vi "Interfaz.vi"() -> ()   [LabVIEW 2023]
uses:
  <vilib>/Instr/_visa.llb/VISA Configure Serial Port (Instr).vi
panel:
  out "Real Altitude":T1(graph)
  out "Y":dbl(knob) scale=-180.0..180.0
  out "Gyro z":T1(graph)
  out "Gyro y":T1(graph)
  out "Gyro x":T1(graph)
  out "X":dbl(knob) scale=-180.0..180.0
  out "Thermometer":dbl(slide) scale=0.0..60.0
  out "salida de x":dbl[](array[numeric])
  out "Input":string
  in  "Select a file":path
  out "Barometer":T1(graph)
  out "Altitude":T1(graph)
  out "Accelerometer Z":cluster{i32[], dbl[]}(graph)
  out "Accelerometer Y":cluster{i32[], dbl[]}(graph)
  out "#Satellites":dbl
  out "Longitude":dbl
  out "Latitude":dbl
  out "Temperature":T1(graph)
  out "Accelerometer X":cluster{i32[], "output array":dbl[]}(graph)
  in  "stop":bool
  in  "Select a communication port":refnum<visa-resource-name>
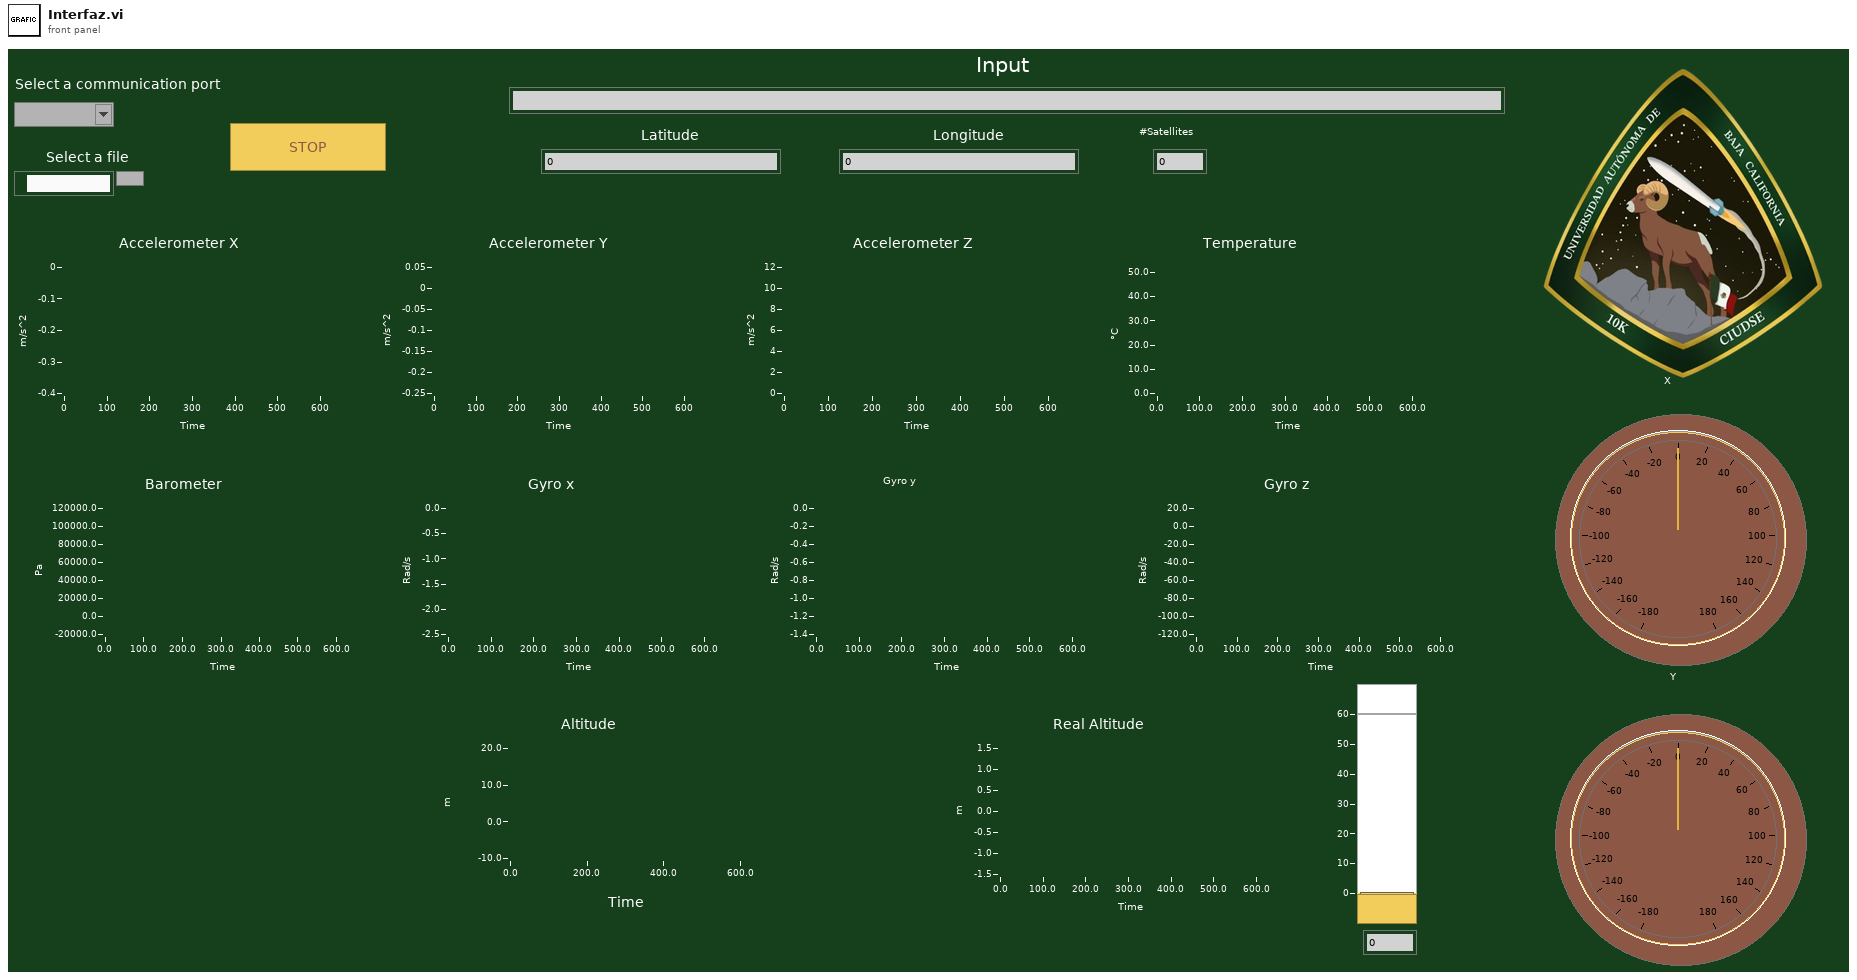
[diagram p1: front panel]
types:
  T1 = cluster{"output array":dbl[], "output array":dbl[]}
  T2 = enum16{"open", "replace", "create", "open or create", "replace or create", "replace or create with confirmation"}
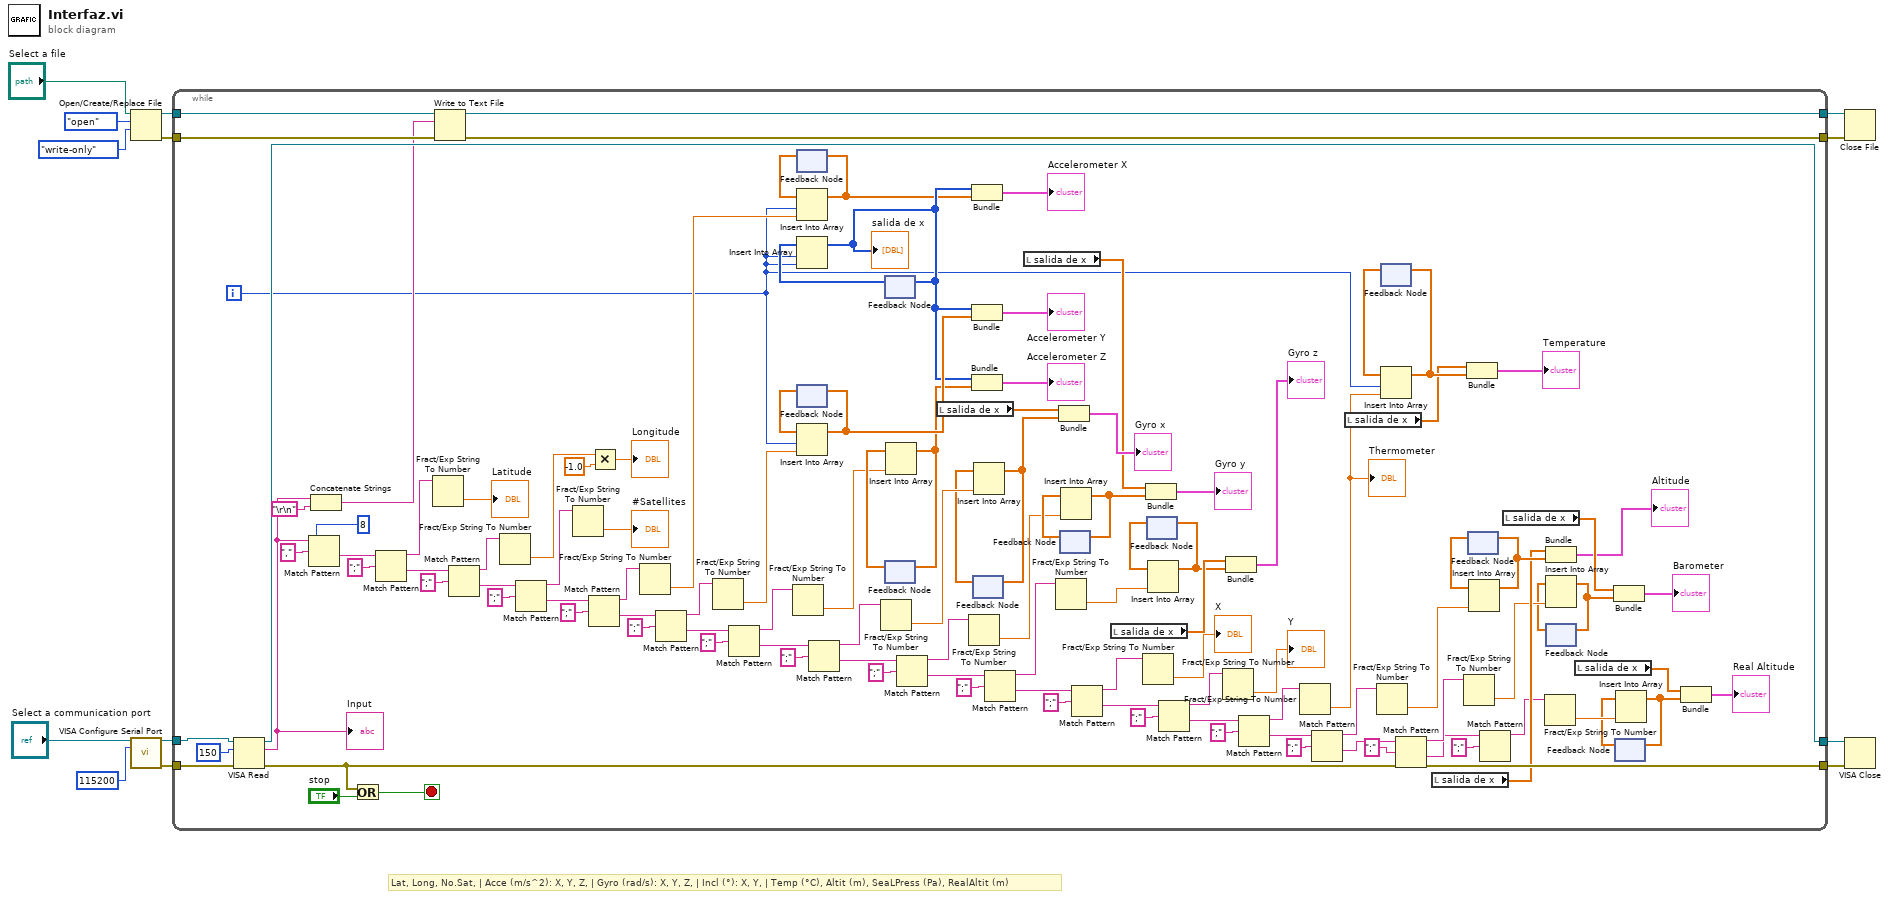
[diagram p0: block diagram]
diagram:
  # "Lat, Long, No.Sat, | Acce (m/s^2): X, Y, Z, | Gyro (rad/s): X, Y, Z, | Incl (°): X, Y, | Temp (°C), Altit (m), SeaLPress (Pa), RealAltit (m)"
  n1 = Open/Create/Replace File(file path (use dialog)="Select a file", operation (0:open)=T2."open", access (0:read/write)=enum16{"read/write", "read-only", "write-only"}."write-only") -> (refnum out=w4:refnum<file>, error out=w1:errorcluster)  [unwired: 3 in, 1 out]
  n2 = call-poly "VISA Configure Serial Port"("VISA resource name"="Select a communication port", "baud rate (9600)"=u32 115200) -> ("VISA resource name out"=w11:refnum<visa-resource-name>, "error out"=w9:errorcluster)  [unwired: 12 in]
  n3 = while {
    tunnel: w11 -> [w131]
    tunnel: [w130] -> w10
    tunnel: w9 -> [w129]
    tunnel: [w126] -> w8
    tunnel: w4 -> [w123]
    tunnel: [w122] -> w3
    tunnel: [w121] -> w2
    tunnel: w1 -> [w120]
    i -> [w33]
    stop <- w125 stop-if-true
    n4 = VISA Read(VISA resource name=w131, byte count=u32 150, error in (no error)=w129) -> (VISA resource name out=w130:refnum<visa-resource-name>, read buffer=w117:string, error out=w126:errorcluster)  [unwired: 1 out]
    "Input" <- w117
    n5 = Match Pattern(string=w117, regular expression=",", offset (0)=8) -> (after substring=w28:string)  [unwired: 3 out]
    n6 = Concatenate Strings(w117, "\r\n") -> (w118:string)
    n7 = Or(x=w126, y="stop") -> (x .or. y?=w125:bool)
    n8 = Match Pattern(string=w28, regular expression=";") -> (before substring=w70:string, after substring=w64:string)  [unwired: 1 in, 2 out]
    n9 = Fract/Exp String To Number(string=w70) -> (number=→"Latitude":dbl)  [unwired: 3 in, 1 out]
    n10 = Write to Text File(file (use dialog)=w123, text=w118, error in=w120) -> (refnum out=w122:refnum<file>, error out=w121:errorcluster)  [unwired: 1 in, 1 out]
    n11 = Match Pattern(string=w64, regular expression=";") -> (before substring=w68:string, after substring=w62:string)  [unwired: 1 in, 2 out]
    n12 = Fract/Exp String To Number(string=w68) -> (number=w41:dbl)  [unwired: 3 in, 1 out]
    n13 = Match Pattern(string=w62, regular expression=";") -> (before substring=w65:string, after substring=w29:string)  [unwired: 1 in, 2 out]
    n14 = Fract/Exp String To Number(string=w65) -> (number=→"#Satellites":dbl)  [unwired: 3 in, 1 out]
    n15 = Match Pattern(string=w29, regular expression=";") -> (before substring=w31:string, after substring=w30:string)  [unwired: 1 in, 2 out]
    n16 = Multiply(x=w41, y=-1.0) -> (x*y=→"Longitude":dbl)
    n17 = Fract/Exp String To Number(string=w31) -> (number=w36:dbl)  [unwired: 3 in, 1 out]
    n18 = Match Pattern(string=w30, regular expression=";") -> (before substring=w112:string, after substring=w106:string)  [unwired: 1 in, 2 out]
    n19 = Fract/Exp String To Number(string=w112) -> (number=w111:dbl)  [unwired: 3 in, 1 out]
    n20 = Match Pattern(string=w106, regular expression=";") -> (before substring=w108:string, after substring=w100:string)  [unwired: 1 in, 2 out]
    n21 = Fract/Exp String To Number(string=w108) -> (number=w107:dbl)  [unwired: 3 in, 1 out]
    n22 = feedback #1() -> (w35:dbl[])  [unwired: 1 in]
    n23 = Insert Into Array(array=w35, index=w33, new element=w36) -> (w32:dbl[])
    n24 = feedback-in #1(w32) -> ()
    n25 = feedback #2() -> (w113:dbl[])  [unwired: 1 in]
    n26 = Insert Into Array(array=w113, index=w33, new element=w111) -> (w110:dbl[])
    n27 = feedback-in #2(w110) -> ()
    n28 = Match Pattern(string=w100, regular expression=";") -> (before substring=w102:string, after substring=w95:string)  [unwired: 1 in, 2 out]
    n29 = Fract/Exp String To Number(string=w102) -> (number=w53:dbl)  [unwired: 3 in, 1 out]
    n30 = feedback #3() -> (w38:i32[])  [unwired: 1 in]
    n31 = Insert Into Array(array=w38, index=w33, new element=w33) -> (w37:i32[])
    "salida de x" <- w37
    n32 = feedback-in #3(w37) -> ()
    n33 = feedback #4() -> (w109:dbl[])  [unwired: 1 in]
    n34 = Insert Into Array(array=w109, new element=w107) -> (w105:dbl[])  [unwired: 1 in]
    n35 = feedback-in #4(w105) -> ()
    n36 = Match Pattern(string=w95, regular expression=";") -> (before substring=w99:string, after substring=w94:string)  [unwired: 1 in, 2 out]
    n37 = local read "salida de x"() -> (w55:dbl[])
    n38 = Fract/Exp String To Number(string=w99) -> (number=w43:dbl)  [unwired: 3 in, 1 out]
    n39 = Bundle(w37, w32) -> (→"Accelerometer X":cluster{i32[], dbl[]})  [unwired: 1 in]
    n40 = Bundle(w37, w110) -> (→"Accelerometer Y":cluster{i32[], dbl[]})  [unwired: 1 in]
    n41 = Bundle(w37, w105) -> (→"Accelerometer Z":cluster{i32[], dbl[]})  [unwired: 1 in]
    n42 = feedback #5() -> (w52:dbl[])  [unwired: 1 in]
    n43 = Insert Into Array(array=w52, new element=w53) -> (w54:dbl[])  [unwired: 1 in]
    n44 = feedback-in #5(w54) -> ()
    n45 = Match Pattern(string=w94, regular expression=";") -> (before substring=w97:string, after substring=w91:string)  [unwired: 1 in, 2 out]
    n46 = local read "salida de x"() -> (w49:dbl[])
    n47 = Fract/Exp String To Number(string=w97) -> (number=w42:dbl)  [unwired: 3 in, 1 out]
    n48 = Bundle("salida de x"=w55, w54) -> (→"Gyro x":cluster{"salida de x":dbl[], dbl[]})  [unwired: 1 in]
    n49 = feedback #6() -> (w51:dbl[])  [unwired: 1 in]
    n50 = Insert Into Array(array=w51, new element=w43) -> (w50:dbl[])  [unwired: 1 in]
    n51 = feedback-in #6(w50) -> ()
    n52 = Match Pattern(string=w91, regular expression=";") -> (before substring=w93:string, after substring=w24:string)  [unwired: 1 in, 2 out]
    n53 = local read "salida de x"() -> (w46:dbl[])
    n54 = Fract/Exp String To Number(string=w93) -> (number=→"X":dbl)  [unwired: 3 in, 1 out]
    n55 = Bundle("salida de x"=w49, w50) -> (→"Gyro y":cluster{"salida de x":dbl[], dbl[]})  [unwired: 1 in]
    n56 = feedback #7() -> (w44:dbl[])  [unwired: 1 in]
    n57 = Insert Into Array(array=w44, new element=w42) -> (w45:dbl[])  [unwired: 1 in]
    n58 = feedback-in #7(w45) -> ()
    n59 = Match Pattern(string=w24, regular expression=";") -> (before substring=w27:string, after substring=w23:string)  [unwired: 1 in, 2 out]
    n60 = Fract/Exp String To Number(string=w27) -> (number=→"Y":dbl)  [unwired: 3 in, 1 out]
    n61 = Bundle("salida de x"=w46, w45) -> (→"Gyro z":cluster{"salida de x":dbl[], dbl[]})  [unwired: 1 in]
    n62 = Match Pattern(string=w23, regular expression=";") -> (before substring=w90:string, after substring=w79:string)  [unwired: 1 in, 2 out]
    n63 = Fract/Exp String To Number(string=w90) -> (number=w58:dbl)  [unwired: 3 in, 1 out]
    "Thermometer" <- w58
    n64 = Match Pattern(string=w79, regular expression=";") -> (before substring=w81:string, after substring=w72:string)  [unwired: 1 in, 2 out]
    n65 = local read "salida de x"() -> (w86:dbl[])
    n66 = Fract/Exp String To Number(string=w81) -> (number=w82:dbl)  [unwired: 3 in, 1 out]
    n67 = feedback #8() -> (w87:dbl[])  [unwired: 1 in]
    n68 = Insert Into Array(array=w87, index=w33, new element=w58) -> (w88:dbl[])
    n69 = feedback-in #8(w88) -> ()
    n70 = Match Pattern(string=w72, regular expression=";") -> (before substring=w77:string, after substring=w15:string)  [unwired: 1 in, 2 out]
    n71 = local read "salida de x"() -> (w80:dbl[])
    n72 = Fract/Exp String To Number(string=w77) -> (number=w76:dbl)  [unwired: 3 in, 1 out]
    n73 = Bundle("salida de x"=w86, w88) -> (→"Temperature":cluster{"salida de x":dbl[], dbl[]})  [unwired: 1 in]
    n74 = feedback #9() -> (w85:dbl[])  [unwired: 1 in]
    n75 = Insert Into Array(array=w85, new element=w82) -> (w84:dbl[])  [unwired: 1 in]
    n76 = feedback-in #9(w84) -> ()
    n77 = Match Pattern(string=w15, regular expression=";") -> (before substring=w19:string)  [unwired: 1 in, 3 out]
    n78 = local read "salida de x"() -> (w78:dbl[])
    n79 = Fract/Exp String To Number(string=w19) -> (number=w20:dbl)  [unwired: 3 in, 1 out]
    n80 = Bundle("salida de x"=w80, w84) -> (→"Altitude":cluster{"salida de x":dbl[], dbl[]})  [unwired: 1 in]
    n81 = feedback #10() -> (w73:dbl[])  [unwired: 1 in]
    n82 = Insert Into Array(array=w73, new element=w76) -> (w74:dbl[])  [unwired: 1 in]
    n83 = feedback-in #10(w74) -> ()
    n84 = local read "salida de x"() -> (w18:dbl[])
    n85 = Bundle("salida de x"=w78, w74) -> (→"Barometer":cluster{"salida de x":dbl[], dbl[]})  [unwired: 1 in]
    n86 = feedback #11() -> (w17:dbl[])  [unwired: 1 in]
    n87 = Insert Into Array(array=w17, new element=w20) -> (w16:dbl[])  [unwired: 1 in]
    n88 = feedback-in #11(w16) -> ()
    n89 = Bundle("salida de x"=w18, w16) -> (→"Real Altitude":cluster{"salida de x":dbl[], dbl[]})  [unwired: 1 in]
  }
  n90 = Close File(refnum=w3, error in=w2) -> ()  [unwired: 2 out]
  n91 = VISA Close(VISA resource name=w10, error in (no error)=w8) -> ()  [unwired: 1 out]
